vi "Acquire.vi"(8 "error in":errorcluster, 11 "StellarNetSpectrometer in":refnum<class "StellarNetSpectrometer.lvclass">) -> (0 "error out":errorcluster, 3 "StellarNetSpectrometer out":refnum<class "StellarNetSpectrometer.lvclass">)   [LabVIEW 2013]
uses:
  StellarNetSpecAcquisitionClass/StellarNetSpecAcquisition.lvclass
  StellarNetSpectrometer.lvclass
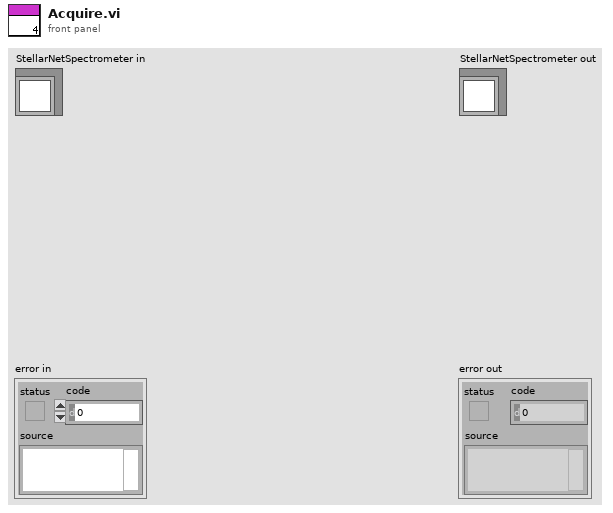
[diagram p1: front panel]
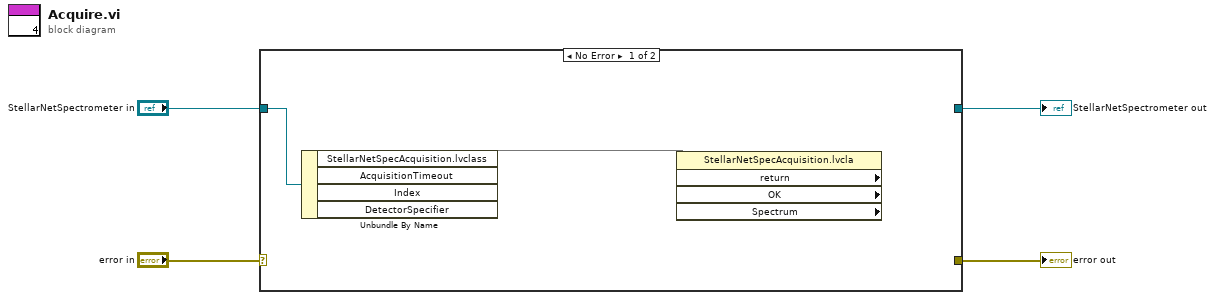
[diagram p0: block diagram]
diagram:
  n1 = case shown="No Error" "error in" {
    selector: "error in" -> [w12 w17]
    tunnel: [w11 w17] -> w3
    tunnel: [w9 w16] -> w1
    tunnel: "StellarNetSpectrometer in" -> [w10 w16]
    frame No Error {
      n2 = Unbundle By Name(w10) -> ("StellarNetSpecAcquisition.lvclass"=w5, "AcquisitionTimeout"=w15, "Index"=w14, "DetectorSpecifier"=w13)
      n3 = property class="StellarNetSpecAcquisition.lvcla"(reference=w5) -> ("return"=w8:i32, "OK"=w7:bool, "Spectrum"=w6:sgl[])  [unwired: 1 in, 2 out]
    }
    frame Error {
    }
  }
  "error out" <- w3
  "StellarNetSpectrometer out" <- w1
